vi "CreatePublicEvents.vi"(8 "error in (no error)":errorcluster, 11 "EmbeddedSMO":refnum<class "SMO.UI.Embedded.lvclass">) -> (0 "error out":errorcluster, 3 "EmbeddedSMO out":refnum<class "SMO.UI.Embedded.lvclass">)   [LabVIEW 2019, in "SMO.UI.Embedded.lvclass"]
doc: "---------------------------------------------------------------\nJKI State Machine Objects™\nhttp://jki.net/state-machine-objects/\nCopyright (C) 2005-2015, JKI <info@jki.net>\nALL RIGHTS RESERVEDJKI State Machine Objects (SMO) 1.0.0.4\nJKI - JKI\nCopyright (c) 2015, JKI"
uses:
  SMO.UI.Embedded.lvclass
  Typedefs/PublicEvents--SMO.UI.Embedded.ReadyForInfo.ctl
  Typedefs/PublicEvents--SMO.UI.Embedded.UIState.ctl
  Typedefs/UI State.ctl
  SMO.UI.Embedded.lvclass/SMO.UI.Embedded.ctl
  <vilib>/JKI/JKI SMO/SMO.UI/SMO.UI.lvclass
panel:
  # "For instructions on how to use the JKI State Machine Objects, examples and video tutorials, visit:\nhttp://jki.net/state-machine-objects/\n\nJKI State Machine Objects™\nhttp://jki.net/state-machine-objects/\nCopyright (C) 2005-2015, JKI <info@jki.net>\nALL RIGHTS RESERVED"
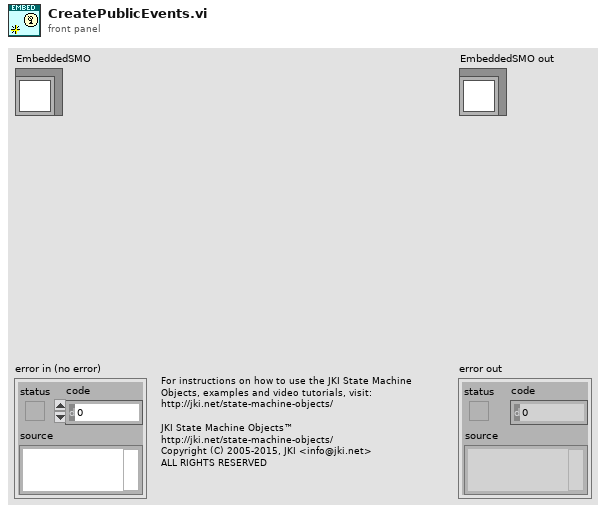
[diagram p1: front panel]
types:
  T1 = typedef "SMO.UI.Embedded.lvclass/PublicEvents--SMO.UI.Embedded.UIState.ctl" = cluster{"UI State":T2, "GUID":string}
  T2 = typedef "SMO.UI.Embedded.lvclass/UI State.ctl" = enum16{"unknown", "Opened", "Embedded", "Closed"}
  T3 = typedef "SMO.UI.Embedded.lvclass/PublicEvents--SMO.UI.Embedded.ReadyForInfo.ctl" = bool
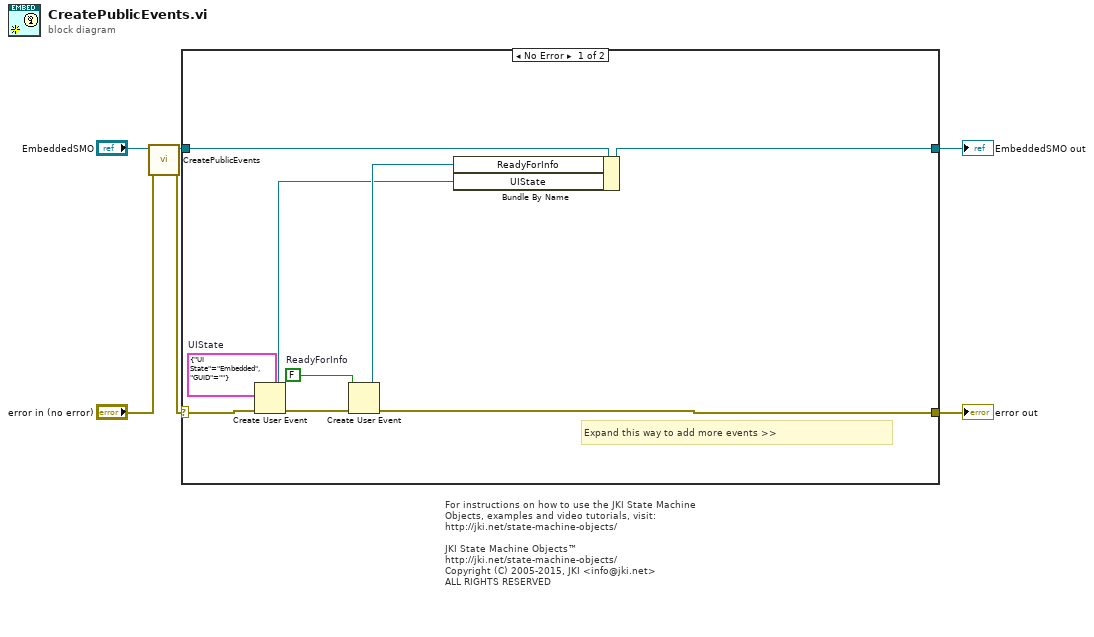
[diagram p0: block diagram]
diagram:
  # "For instructions on how to use the JKI State Machine Objects, examples and video tutorials, visit:\nhttp://jki.net/state-machine-objects/\n\nJKI State Machine Objects™\nhttp://jki.net/state-machine-objects/\nCopyright (C) 2005-2015, JKI <info@jki.net>\nALL RIGHTS RESERVED"
  n1 = call-parent "CreatePublicEvents.vi"("error in (no error)"="error in (no error)", "SMO.UI"="EmbeddedSMO") -> ("error out"=w1:errorcluster, "SMO.UI out"=w3:refnum<class "SMO.UI.Embedded.lvclass">)  [unwired: 8 in]
  n2 = case shown="No Error" w1 {
    selector: w1 -> [w14 w17]
    tunnel: [w12 w17] -> w5
    tunnel: [w13 w16] -> w6
    tunnel: w3 -> [w15 w16]
    frame No Error {
      w8 = T1 {"UI State"=enum."Embedded", "GUID"=""}  # UIState
      w11 = T3 FALSE  # ReadyForInfo
      # "Expand this way to add more events >>"
      n3 = Create User Event(user event datatype=w8, error in=w14) -> (user event=w7:refnum<user-event>, error out=w9:errorcluster)
      n4 = Create User Event(user event datatype=w11, error in=w9) -> (user event=w10:refnum<user-event>, error out=w12:errorcluster)
      n5 = Bundle By Name(cluster=w15, "ReadyForInfo"=w10, "UIState"=w7) -> (w13:refnum<class "SMO.UI.Embedded.lvclass">)
    }
    frame Error {
    }
  }
  "error out" <- w5
  "EmbeddedSMO out" <- w6
